vi "Read RT FIFO.vi"(7 "fifo options":T1, 8 "error in (no error)":errorcluster, 9 "timeout in ms (0)":i32, 11 "rt fifo in":refnum<k33>) -> (0 "error out":errorcluster, 1 "empty?":bool, 2 "element":u8[](array[numeric]), 3 "rt fifo out":refnum<k33>, 4 "# elements":u32)   [LabVIEW 2019, in "DSF Core.lvlib" / "Interface.lvclass"]
uses:
  Interface.lvclass
  Typedefs/DSF FIFO Options.ctl
  Framework/Framework.lvclass
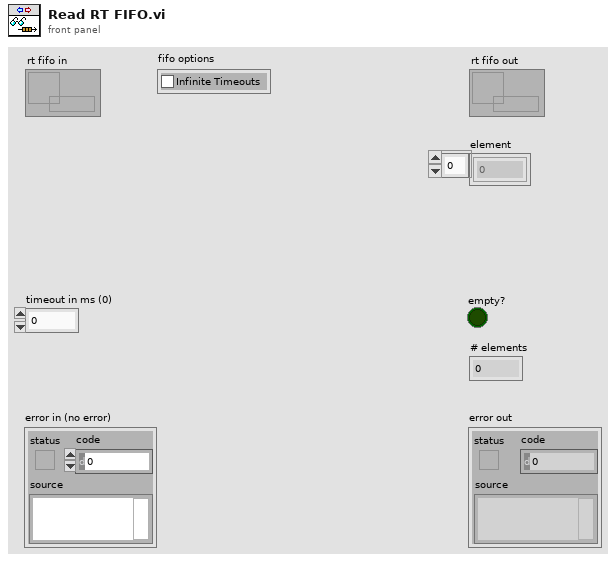
[diagram p1: front panel]
types:
  T1 = typedef "DSF Core.lvlib/Framework.lvclass/DSF FIFO Options.ctl" = cluster{"Infinite Timeouts":bool}
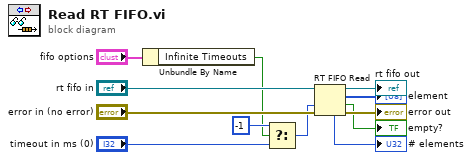
[diagram p0: block diagram]
diagram:
  n1 = Unbundle By Name("fifo options") -> ("Infinite Timeouts"=w2:bool)
  n2 = Select(t=-1, s=w2, f="timeout in ms (0)") -> (s? t:f=w4:i32)
  n3 = RT FIFO Read(0:"rt fifo in", 2:w4, 3:"error in (no error)") -> (7:→"# elements":u32, 8:→"rt fifo out":refnum<k33>, 9:→"element":u8[], 10:→"empty?":bool, 11:→"error out":errorcluster)  [unwired: 1 in]
